vi "Collect_Info_updated.vi"(5 "HART ports":refnum<visa-resource-name>[](array[refnum]), 7 "485 Ports":refnum<visa-resource-name>[](array[refnum]), 10 "MODBUS Serial Parameters":T8={"Mode"=enum."RTU", "Default Slave Address"=111, "MODBUS timeout"=1000, "Baud Rate"=38400, "Parity"=0, "Flow Control"=0} {"Flow Control" items=["None", "XON/XOFF", "RTS/CTS", "XON/XOFF & RTS/CTS", "DTR/DSR", "XON/XOFF & DTR/DSR"]; "Parity" items=["None", "Odd", "Even", "Mark", "Space"]}) -> (1 "Read Completed":bool, 2 "Information":T9, 3 "Byte order":T2(ring))   [LabVIEW 2016]
uses:
  Controls/Flow Tube Material.ctl
  Controls/mass flow unit codes.ctl
  Controls/Density Unit codes.ctl
  Controls/Temperature units.ctl
  Controls/Flow direction codes.ctl
  Controls/Information_tab_type.ctl
  OPC Server/MODBUS/MODBUS parameters type.ctl
  <vilib>/DeviceNet/VIAPI/subVIs/DnetIntfConfig.ctl
  OPC Server/Typedef/Array_of_Comm_mode_and_address_types.ctl
  OPC Server/Typedef/Comm_mode_and_address_type.ctl
  OPC Server/Typedef/Comm_mode_type_combo.ctl
  types/Control_EXIT.ctl
  Controls/ctrlCollectInfoStates.ctl
  Controls/ctrlCollectInfoData.ctl
  OPC Server/Protocol Class/Protocol.lvclass
  OPC Server/Typedef/comm_variable_definition.ctl
  OPC Server/MASTER_OPC.ctl
  OPC Server/Typedef/event var.ctl
  OPC Server/Typedef/Comm ui action type.ctl
  OPC Server/Typedef/Comm_State_enum.ctl
  OPC Server/Typedef/state var.ctl
  <vilib>/Utility/miscctls.llb/LVPointTypeDef.ctl
  OPC Server/MODBUS/MODBUS Class/MODBUS.lvclass
  C:/Applications/Blackbox_US-Rabi--master/OPC Server/Protocol Class/Protocol.lvclass
  OPC Server/HART/HART Class/HART.lvclass
  OPC Server/Profibus/Profibus Class/Profibus.lvclass
  OPC Server/DeviceNET/DeviceNET Class/DeviceNET.lvclass
  OPC Server/Typedef/Protocol_enum_type.ctl
  <vilib>/DeviceNet/DeviceNetLIB.lvlib
panel:
  in  "Exit":T1
  in  "MDOT":string="H2O"
  in  "Meter inlet static pressure (psia)":dbl
  in  "Fluid":string="H2O"
  in  "Product code*":string
  in  "Order number":string
  in  "Status *":enum32{"As found", "As left"}(radio)
  in  "Ref meter serial number*":string
  in  "Technician Name*":string
  in  "Customer Address":string
  in  "Customer Name":string
  in  "Done":bool
  out "status":bool
  in  "Protocol selection\n(appended)":T3=[{"address"=111, "Mode"=0}, {"address"=0, "Mode"=2}] {"Mode" items=["MODBUS", "HART", ""]}
  in  "Interface Name":T6(ring)
  in  "DeviceNet Interface Configuration":T7={"interface MAC ID"=0, "baud rate"=enum."500000", "poll mode"=enum."Automatic"} {"interface MAC ID" max=63 step=1}
  in  "Profibus Baud rate":i32(listbox)=6
  in  "Profibus ResourceName":refnum<visa-resource-name>="PXI5::11::INSTR"
  in  "Read":bool
  in  "Test Comments":string
  out "Test date and time":string
  out "Meter Zero":string
  in  "Meter Nominal Flow Rate (kg/min)*":string
  in  "Meter Density Repeatability":string
  in  "Meter Density Accuracy":string
  in  "Meter Zero Stability (kg/min) *":string
  in  "Meter flow repeatability":string
  in  "Meter flow accuracy (%) *":string
  out "Frequency span":string
  out "Frequency flow rate":string
  out "Flow direction":T10 items=["Forward flow only", "Reverse flow only", "Bidirectiona flow", "Absolute forward/reverse", "Negate/Forward only", "Negate/Bidirectional"]
  out "Mass flow damping":string
  out "Mass flow cutoff":string
  out "Temperature Units":T11 items=["Degrees Celsius"=32, "Degrees Fahrenheit"=33, "Degrees Rankine"=34, "Degrees Kelvin"=35, ""=0]
  out "Density units":T12 items=["Specific gravity units"=90, "Grams/cubic centimeter"=91, "Kg/cubic meter"=92, "Pounds/US gallon"=93, "Pounds/cubic foot"=94, "Grams/milliliter"=95, "Kg/liter"=96, "Pounds/cubic inch"=98, "Short tons/cubic yard"=99, "Degrees Baume (heavy)"=102, "Degrees Baume (light)"=103, "Degrees API"=104]
  out "Mass flow units":T13 items=["Grams/second"=70, "Grams/minute"=71, "Grams/hour"=72, "Kg/second"=73, "Kg/minute"=74, "Kg/hour"=75, "Kg/day"=76, "Metric tons/minute"=77, "Metric tons/hour"=78, "Metric tons/day"=79, "Pounds/second"=80, "Pounds/minute"=81, "Pounds/hour"=82, "Pounds/day"=83, "Short tons/minute"=84, "Short tons/hour"=85, "Short tons/day"=86, "Long tons/hour"=87, "Long tons/day"=88, "Special"=253]
  out "Transmitter Model":string
  in  "Sensor Model #":string
  in  "Transmitter Serial Number":string
  out "Density Temp Coeff":string
  out "FD":string
  out "K2":string
  out "K1":string
  out "D2":string
  out "D1":string
  out "FCF":string
  in  "Temp Rating":string
  in  "Pressure Rating":string
  out "Sensor Serial Number":string
  out "Flow Tube Material":T14 items=["Hastelloy C-22"=3, "Monel"=4, "Tantalum"=5, "Titanium"=6, "316L Stainless Steel"=19, "Inconel"=23, "Unknown"=252, "Special"=253]
  in  "Size":string
  # "Customer Information"
  # "*Required"
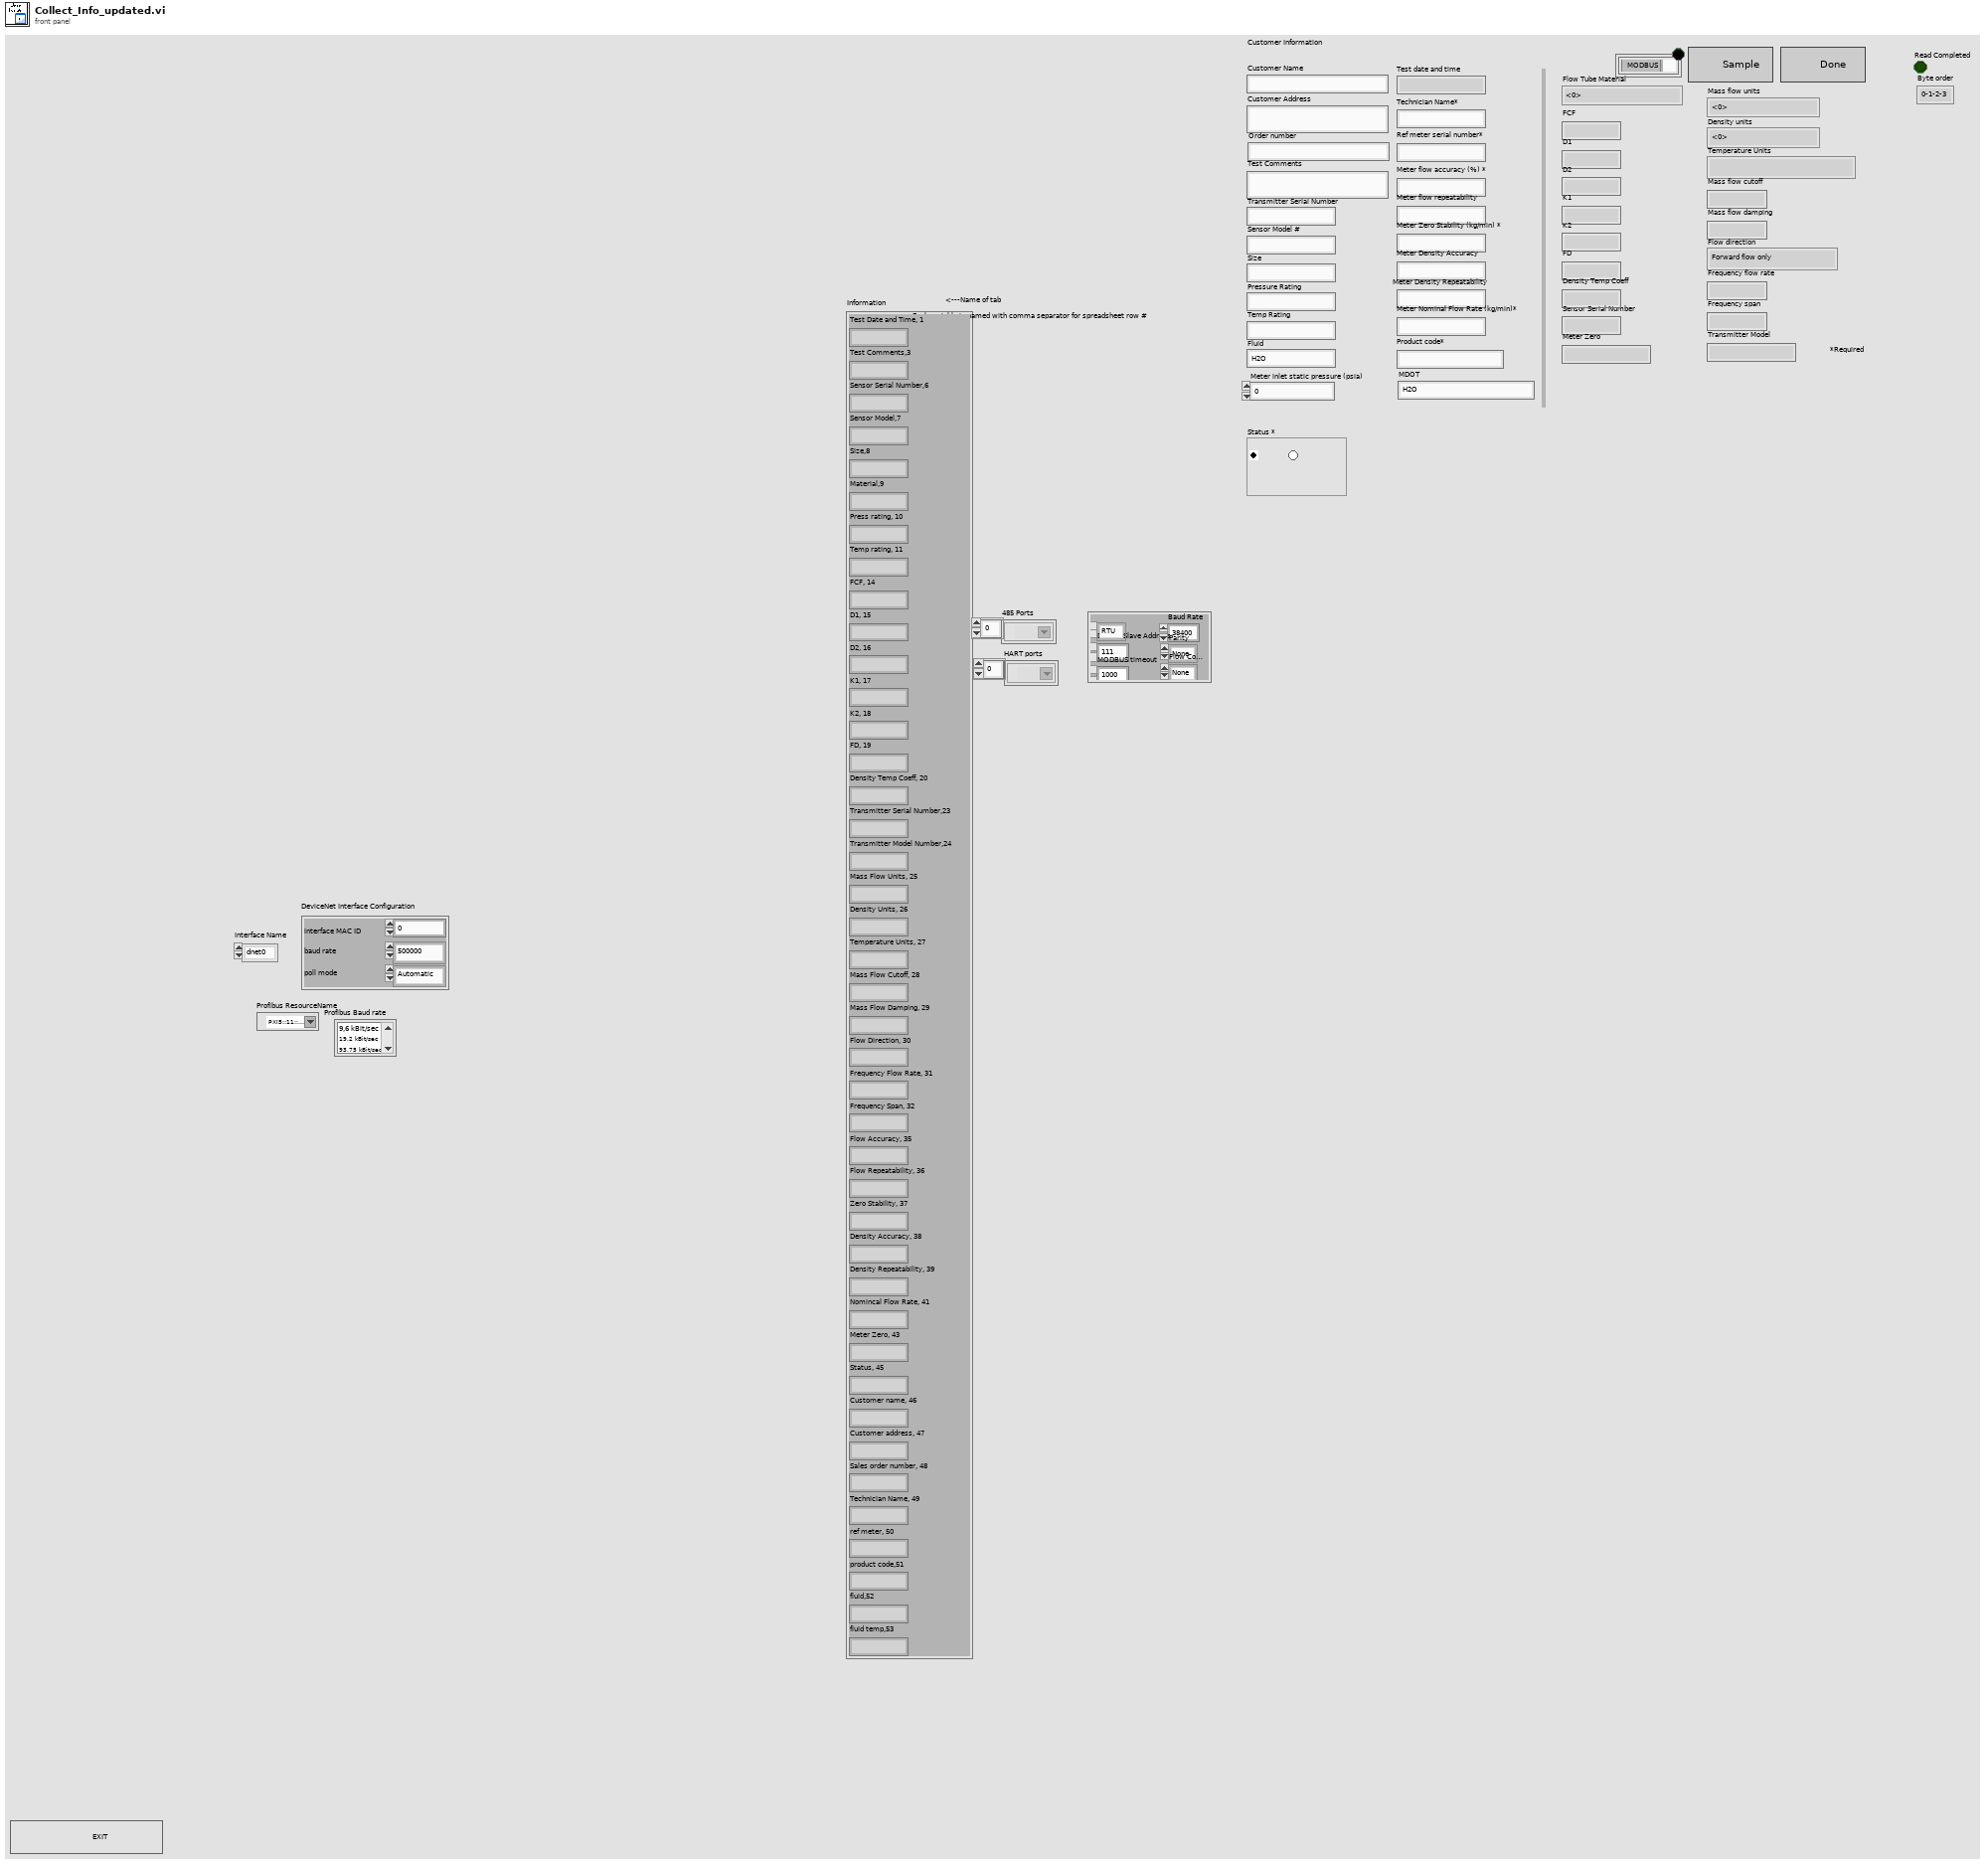
[diagram p1: front panel]
types:
  T1 = typedef "Control_EXIT.ctl" = bool
  T2 = enum16{"0-1-2-3", "2-3-0-1", "1-0-3-2", "3-2-1-0"}
  T3 = typedef "Array_of_Comm_mode_and_address_types.ctl" = T4[]
  T4 = typedef "Comm_mode_and_address_type.ctl" = cluster{"address":i32, "Mode":T5}
  T5 = typedef "Comm_mode_type_combo.ctl" = u16
  T6 = enum16{"dnet0", "dnet1", "dnet2", "dnet3", "dnet4", "dnet5", "dnet6", "dnet7", "dnet8", "dnet9", "dnet10", "dnet11", "dnet12", "dnet13", "dnet14", "dnet15", "dnet16", "dnet17", "dnet18", "dnet19", "dnet20", "dnet21", "dnet22", "dnet23", "dnet24", "dnet25", "dnet26", "dnet27", "dnet28", "dnet29", "dnet30", "dnet31"}
  T7 = typedef "DeviceNetLIB.lvlib/DnetIntfConfig.ctl" = cluster{"interface MAC ID":u32, "baud rate":enum32{"125000", "250000", "500000"}, "poll mode":enum32{"Automatic", "Scanned", "Individual"}}
  T8 = typedef "MODBUS parameters type.ctl" = cluster{"Mode":enum16{"RTU", "ASCII"}, "Default Slave Address":u8, "MODBUS timeout":u32, "Baud Rate":u32, "Parity":u16, "Flow Control":u16}
  T9 = typedef "Information_tab_type.ctl" = cluster{"Test Date and Time, 1":string, "Test Comments,3":string, "Sensor Serial Number,6":string, "Sensor Model,7":string, "Size,8":string, "Material,9":string, "Press rating, 10":string, "Temp rating, 11":string, "FCF, 14":string, "D1, 15":string, "D2, 16":string, "K1, 17":string, "K2, 18":string, "FD, 19":string, "Density Temp Coeff, 20":string, "Transmitter Serial Number,23":string, "Transmitter Model Number,24":string, "Mass Flow Units, 25":string, "Density Units, 26":string, "Temperature Units, 27":string, "Mass Flow Cutoff, 28":string, "Mass Flow Damping, 29":string, "Flow Direction, 30":string, "Frequency Flow Rate, 31":string, "Frequency Span, 32":string, "Flow Accuracy, 35":string, "Flow Repeatability, 36":string, "Zero Stability, 37":string, "Density Accuracy, 38":string, "Density Repeatability, 39":string, "Nomincal Flow Rate, 41":string, "Meter Zero, 43":string, "Status, 45":string, "Customer name, 46":string, "Customer address, 47":string, "Sales order number, 48":string, "Technician Name, 49":string, "ref meter, 50":string, "product code,51":string, "fluid,52":string, "fluid temp,53":string}
  T10 = typedef "Flow direction codes.ctl" = u16
  T11 = typedef "Temperature units.ctl" = u16
  T12 = typedef "Density Unit codes.ctl" = u16
  T13 = typedef "mass flow unit codes.ctl" = u16
  T14 = typedef "Flow Tube Material.ctl" = u16
  T15 = typedef "ctrlCollectInfoData.ctl" = cluster{"HART ports":refnum<visa-resource-name>[], "485 ports":refnum<visa-resource-name>[], "Byte order":enum16{"0-1-2-3", "2-3-0-1", "1-0-3-2", "3-2-1-0"}, "Read Complete?":bool, "ProtocolRef":refnum<vi>, "Data path":path, "ProtocolArray":refnum<class "Protocol.lvclass">[], "Protocol":refnum<class "Protocol.lvclass">, "Comm variable definitions":T16[], "Information":T9}
  T16 = typedef "comm_variable_definition.ctl" = cluster{"General Parameter name":string, "MODBUS Register":i32, "Profibus":cluster{"Friendly name":string, "PA":cluster{"Slot":i32, "Index":i32}, "DP":cluster{"Slot":i32, "Index":i32}, "Tag":string}, "Fieldbus":cluster{"Parameter name":string, "Fieldbus Block":string, "Fieldbus Tag":string}, "data type":enum16{"float", "UINT", "UINT32", "STRING"}, "DeviceNET":cluster{"ClassId":u16, "InstanceId":u16, "AttributeId":u8}, "Cluster":T4, "Length":i32}
  T17 = typedef "ctrlCollectInfoStates.ctl" = enum16{"WaitforEvents", "Init", "Read-Protocol", "Read-CommInfo", "Read-ByteOrder", "Read-FlowTubeMaterial", "Read-FlowCalibFactor", "Read-D1", "Read-D2", "Read-K1", "Read-K2", "Read-FD", "Read-DenTempCoeff", "Read-Srno", "Read-MassFlowUnits", "Read-DensityUnits", "Read-TempUnits", "Read-FlowCutoff", "Read-MassFlowDamping", "Read-FlowDirection", "Read-FreqFlowRate", "Read-FreqSpan", "Read-TransmitterModel", "Read-MeterZero", "ReadComplete", "Done&Close"}
  T18 = typedef "LVPointTypeDef.ctl" = cluster{"Horizontal":i16, "Vertical":i16}
  T19 = typedef "MASTER_OPC.ctl" = cluster{"Main event var":refnum<user-event>, "VIRef":refnum<vi>, "Data path":path, "Reads":i32, "total number of UUT":i32, "FF refnum":cluster{"Handle1":u32, "Handle2":u32}, "FF device id list":string[], "MODBUS resource name":refnum<visa-resource-name>, "MODBUS Serial Parameters":cluster{"Mode":enum16{"RTU", "ASCII"}, "Default Slave Address":u8, "MODBUS timeout":u32, "Baud Rate":u32, "Parity":u16, "Flow Control":u16}, "Profibus resource name":refnum<visa-resource-name>, "Profibus Communication ref.:":u8, "HART resource name":refnum<visa-resource-name>, "HART long addresses (array)":u8[][], "Comm relay session":refnum<k15>, "Comm UI event":refnum<user-event>, "Write Interval (s)":dbl, "DMM_QUEUE":refnum<queue>, "POWER_QUEUE":refnum<queue>, "\nTHERM_QUEUE":refnum<queue>, "\nCOMM_QUEUE":refnum<queue>, "TIMING_QUEUE":refnum<queue>, "MAIN_QUEUE":refnum<queue>, "Log path":path}
  T20 = typedef "Protocol_enum_type.ctl" = enum16{"None", "MODBUS", "HART", "Fieldbus", "Profibus DP", "Profibus PA", "DeviceNET", "USB"}
  T21 = typedef "CS_PB_DPV1_MSAC2_InitiateReqData.ctl" = cluster{"Communication ref.:":u8, "Send timeout:":u16, "Feat. supp. 1:":u8, "Feat. supp. 2:":u8, "Profile feat. supp. 1:":u8, "Profile feat. supp. 2:":u8, "Profile ID number:":u16, "Addional address parameter":cluster{"S-Type":bool, "S-Length:":u8, "D-Type":bool, "D-Length:":u8, "Data:":u8[]}}
  T22 = cluster{"U16":u16, "U32":u32, "float":sgl, "string":string}
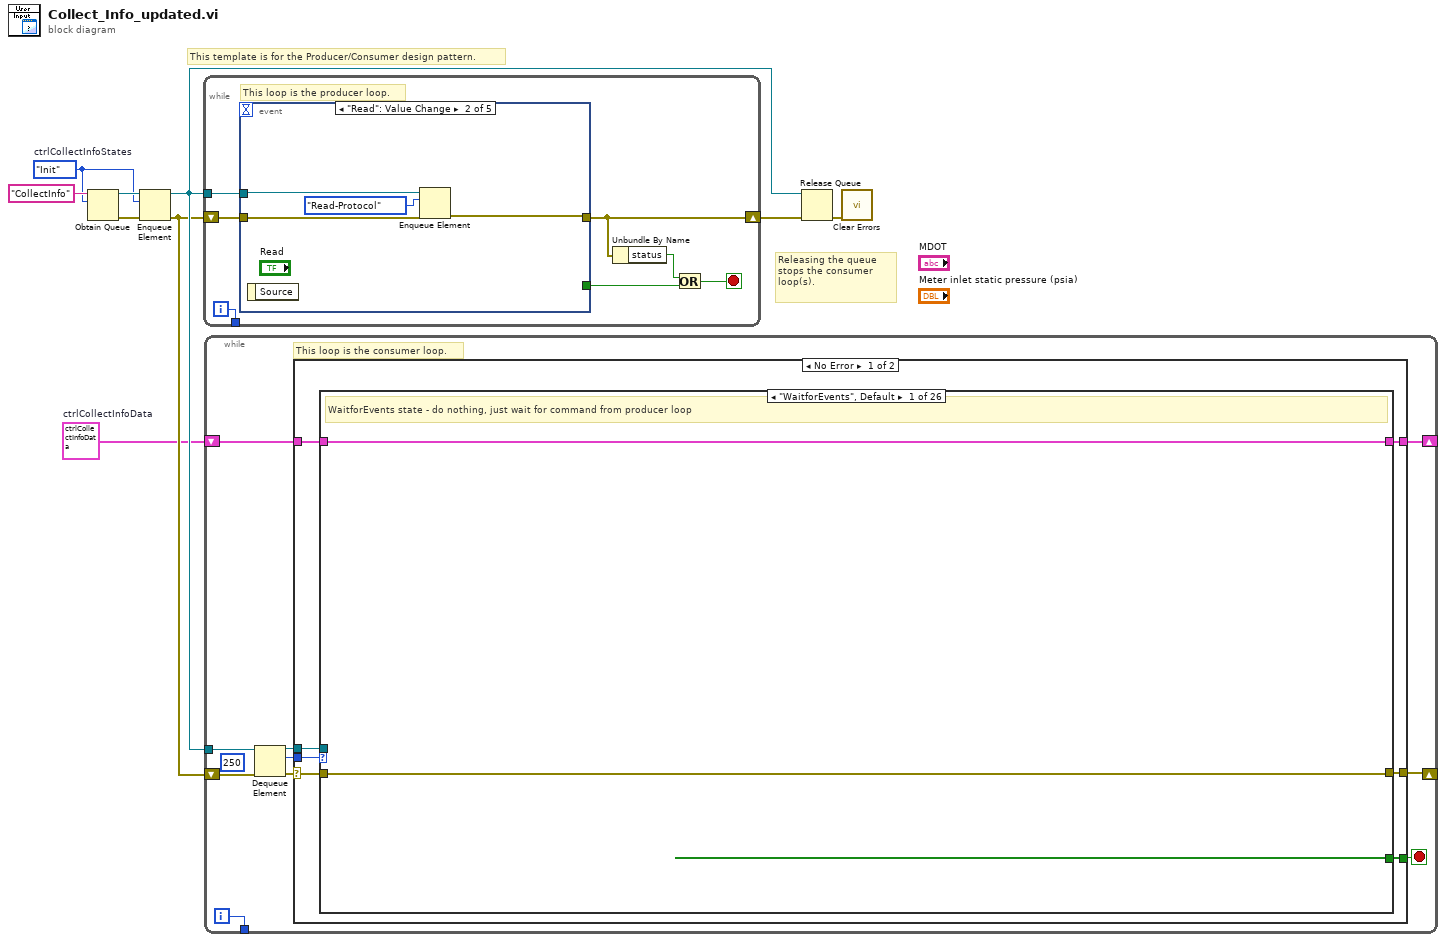
[diagram p0: block diagram]
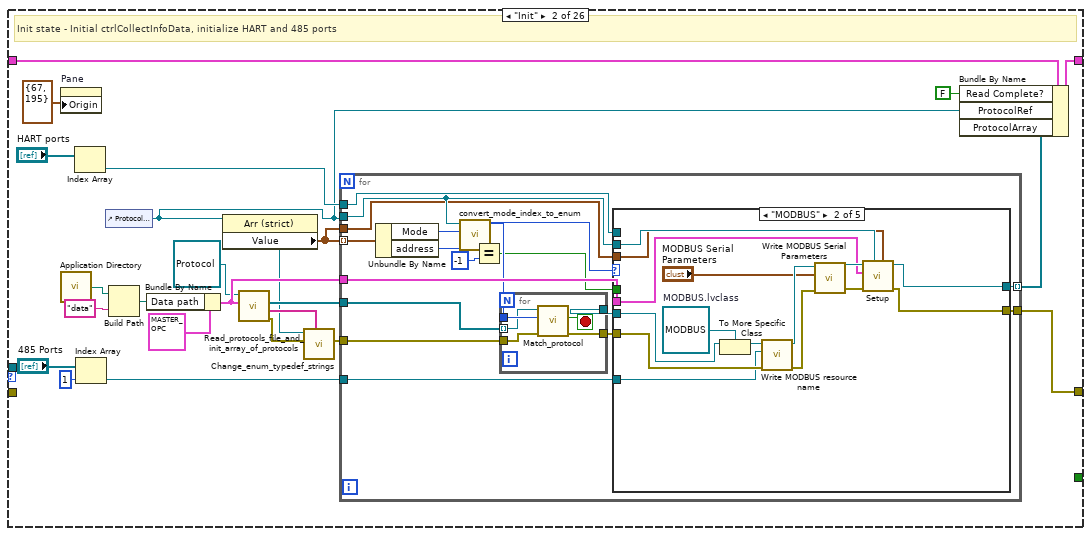
[diagram p2: hidden frame]
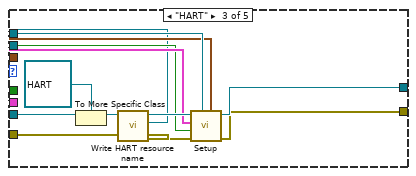
[diagram p4: hidden frame]
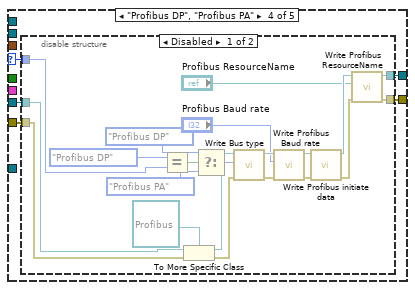
[diagram p5: hidden frame]
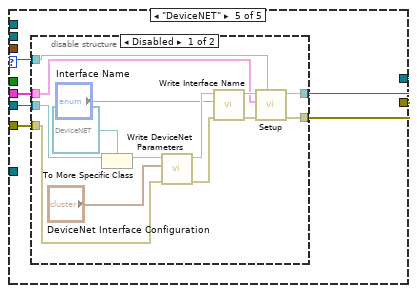
[diagram p7: hidden frame]
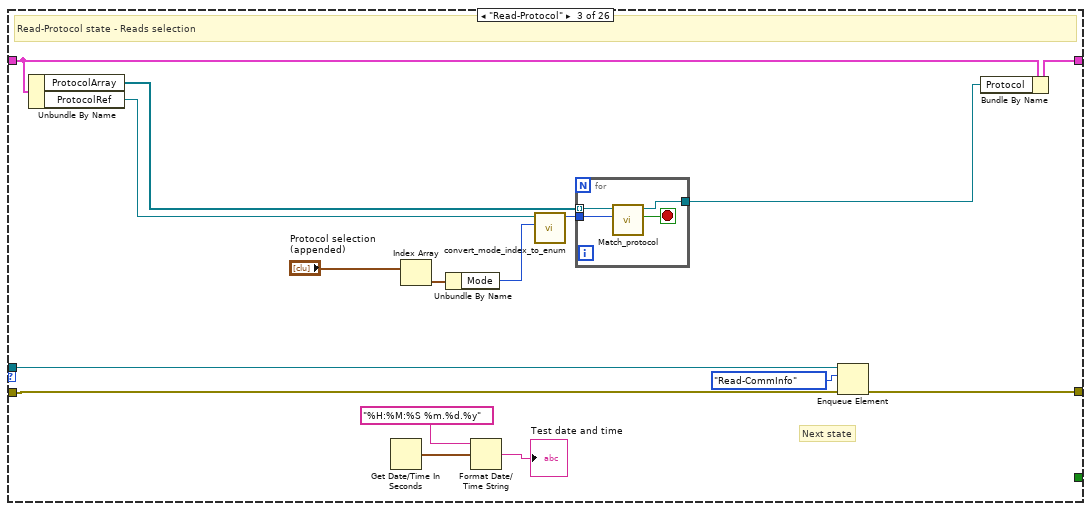
[diagram p9: hidden frame]
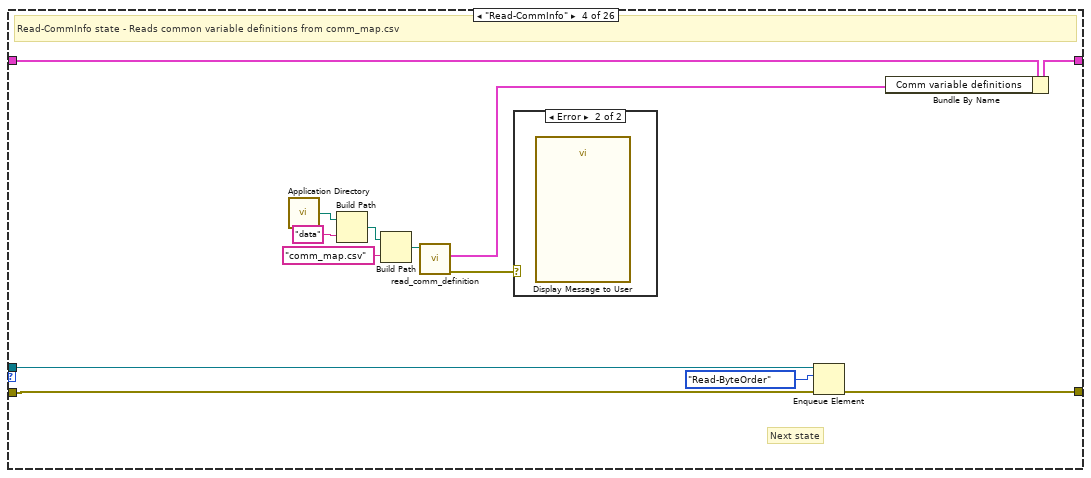
[diagram p10: hidden frame]
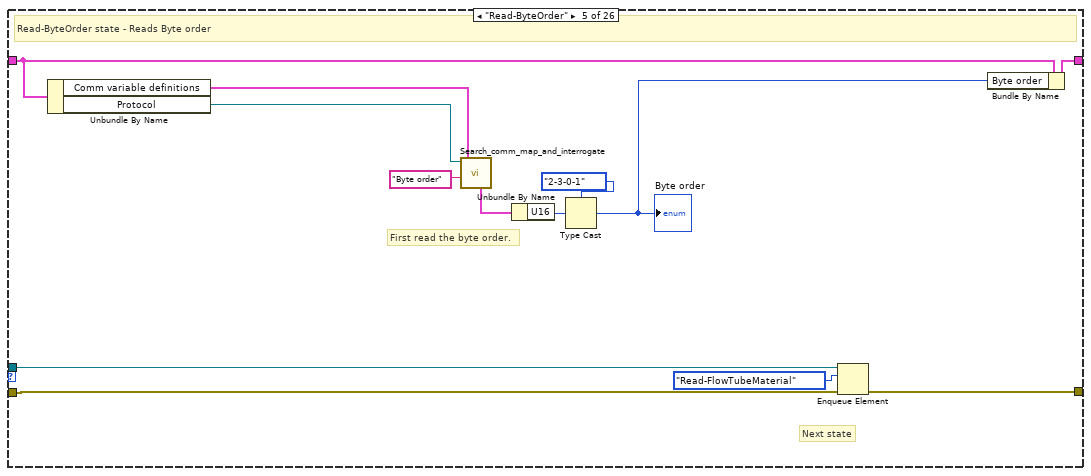
[diagram p12: hidden frame]
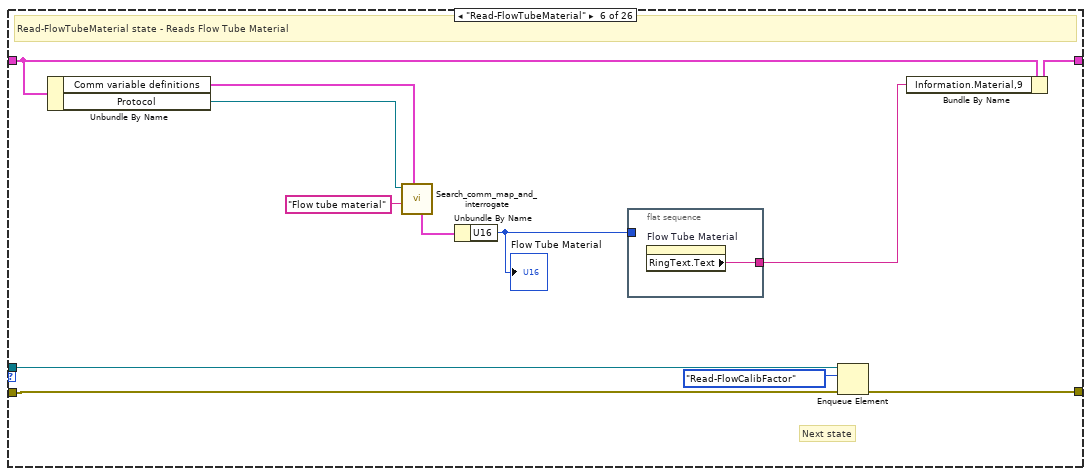
[diagram p13: hidden frame]
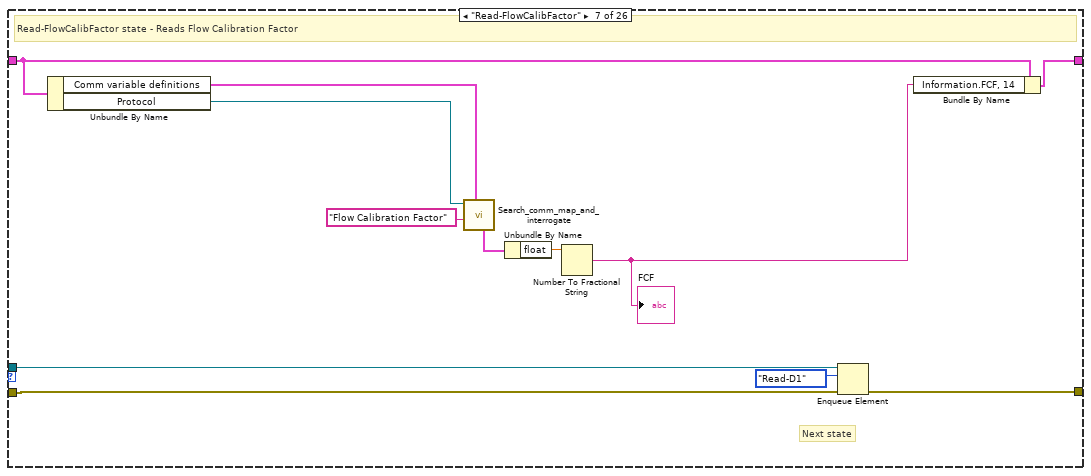
[diagram p14: hidden frame]
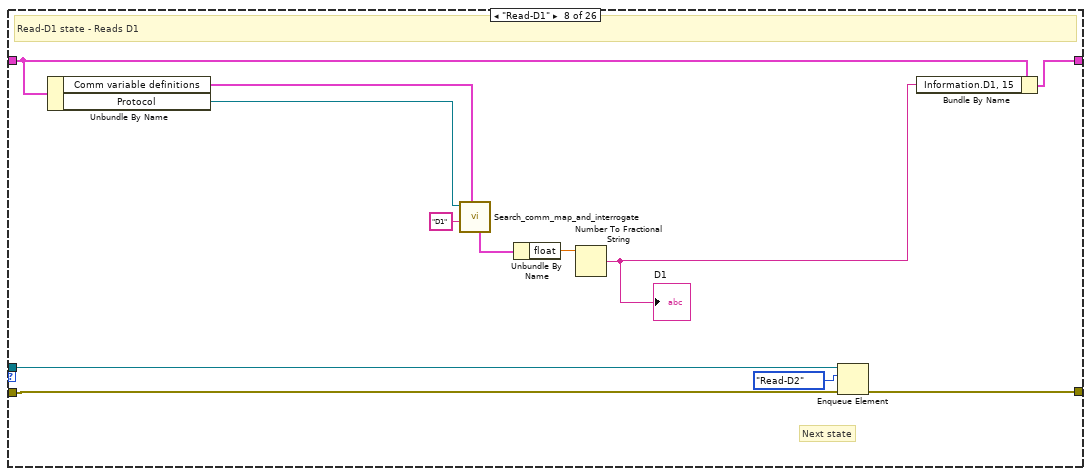
[diagram p15: hidden frame]
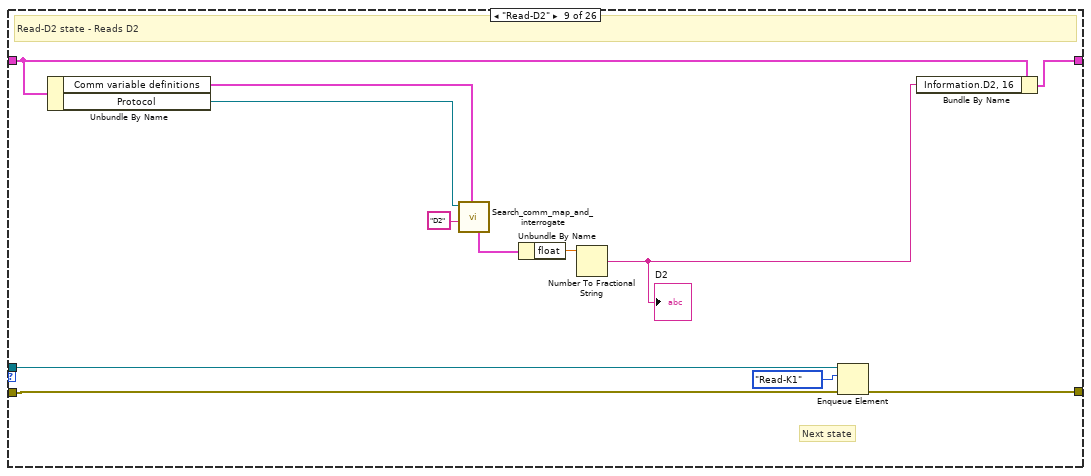
[diagram p16: hidden frame]
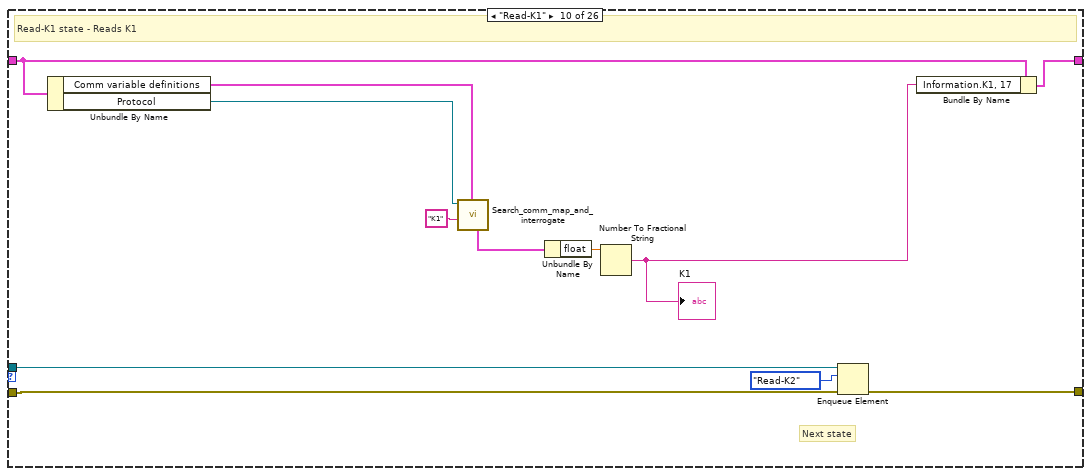
[diagram p17: hidden frame]
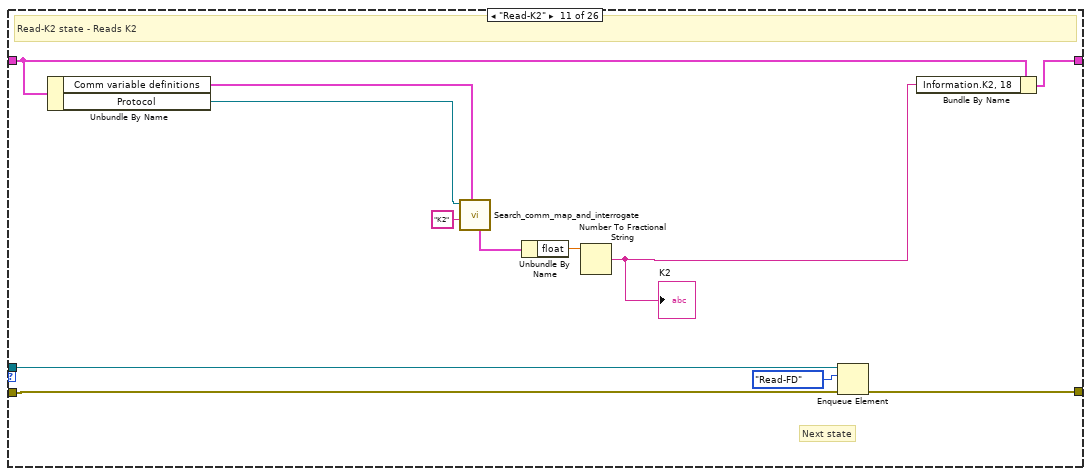
[diagram p18: hidden frame]
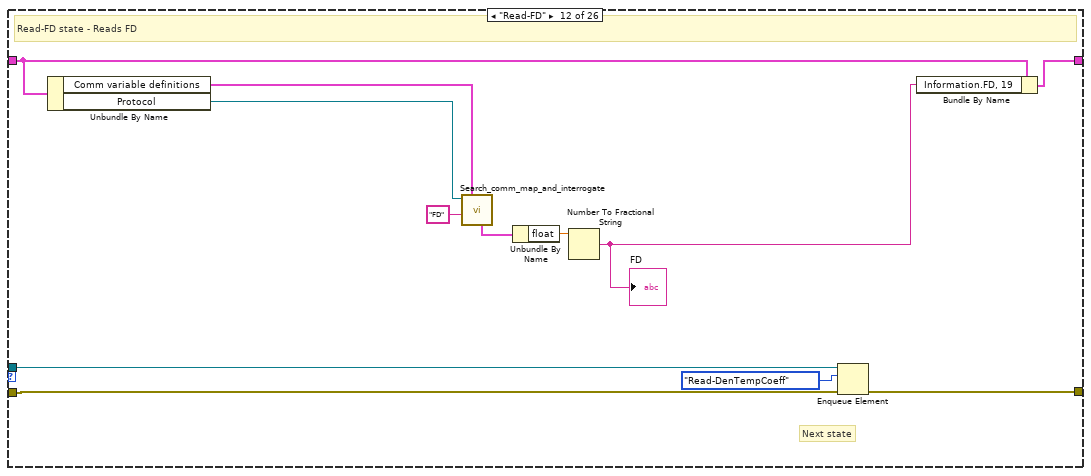
[diagram p19: hidden frame]
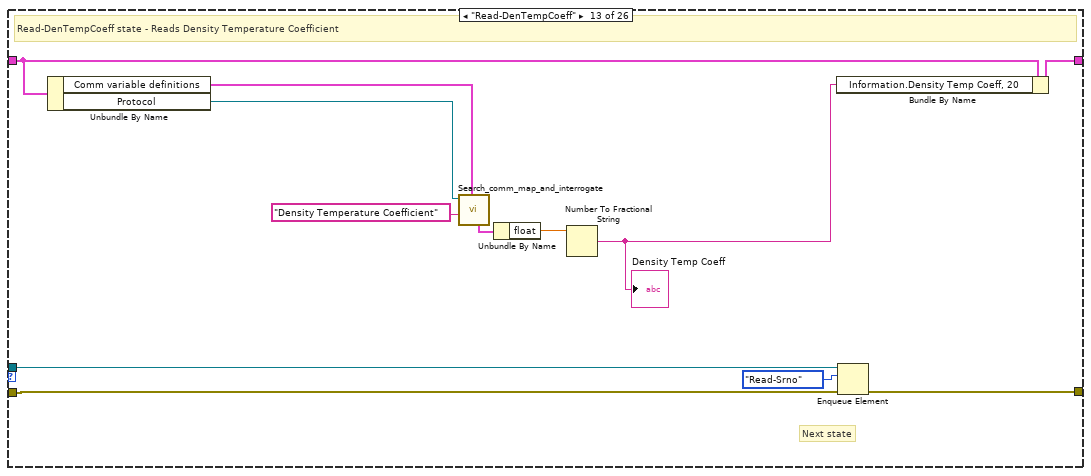
[diagram p20: hidden frame]
diagram:
  w1 = T15 {"HART ports"=[], "485 ports"=[], "Byte order"=enum."0-1-2-3", "Read Complete?"=FALSE, "ProtocolRef"=refnum, "Data path"=path "", "ProtocolArray"=[], "Protocol"=refnum, "Comm variable definitions"=[], "Information"={"Test Date and Time, 1"="", "Test Comments,3"="", "Sensor Serial Number,6"="", "Sensor Model,7"="", "Size,8"="", "Material,9"="", "Press rating, 10"="", "Temp rating, 11"="", "FCF, 14"="", "D1, 15"="", "D2, 16"="", "K1, 17"="", "K2, 18"="", "FD, 19"="", "Density Temp Coeff, 20"="", "Transmitter Serial Number,23"="", "Transmitter Model Number,24"="", "Mass Flow Units, 25"="", "Density Units, 26"="", "Temperature Units, 27"="", "Mass Flow Cutoff, 28"="", "Mass Flow Damping, 29"="", "Flow Direction, 30"="", "Frequency Flow Rate, 31"="", "Frequency Span, 32"="", "Flow Accuracy, 35"="", "Flow Repeatability, 36"="", "Zero Stability, 37"="", "Density Accuracy, 38"="", "Density Repeatability, 39"="", "Nomincal Flow Rate, 41"="", "Meter Zero, 43"="", "Status, 45"="", "Customer name, 46"="", "Customer address, 47"="", "Sales order number, 48"="", "Technician Name, 49"="", "ref meter, 50"="", "product code,51"="", "fluid,52"="", "fluid temp,53"=""}}  # ctrlCollectInfoData
  w2 = ctrlCollectInfoStates."Init"  # ctrlCollectInfoStates
  # "This template is for the Producer/Consumer design pattern."
  # "Releasing the queue stops the consumer loop(s)."
  n1 = Obtain Queue(name (unnamed)="CollectInfo", element data type=w2) -> (queue out=w9:refnum<queue>, error out=w6:errorcluster)  [unwired: 3 in, 1 out]
  n2 = Enqueue Element(queue=w9, element=w2, error in (no error)=w6) -> (queue out=w4:refnum<queue>, error out=w3:errorcluster)  [unwired: 1 in, 1 out]
  n3 = while {
    tunnel: w4 -> [w16]
    tunnel: [w15] -> _
    shift-right: [w11] -> w5
    shift-left: w3 -> [w14]
    i -> [w15]
    stop <- w12 stop-if-true
    # "This loop is the producer loop."
    n4 = event shown="[1] \"Read\": Value Change" {
      selector: _ -> [_ _ _ _ _]
      dyn-events: _ -> [_ _ _ _ _]
      timeout: _ -> [_ _ _ _ _]
      tunnel: w16 -> [w17 w22 w26 _ _]
      tunnel: w14 -> [w20 w24 w29 w34 w39]
      tunnel: [w19 w23 w28 w34 w39] -> w11
      tunnel: [_ _ TRUE ("T button?") w31 w35] -> w10
      event Value Change {
        n5 = event-data() -> ()  [unwired: 1 in, 1 out]
        n6 = Enqueue Element(queue=w17, element=ctrlCollectInfoStates."Init" ("ctrlCollectInfoStates"), error in (no error)=w20) -> (error out=w19:errorcluster)  [unwired: 1 in, 2 out]
      }
      event "Read": Value Change {
        n7 = event-data() -> ()  [unwired: 1 in, 1 out]
        n8 = Enqueue Element(queue=w22, element=ctrlCollectInfoStates."Read-Protocol" ("ctrlCollectInfoStates"), error in (no error)=w24) -> (error out=w23:errorcluster)  [unwired: 1 in, 2 out]
      }
      event "Done": Value Change {
        n9 = event-data() -> ()  [unwired: 1 in, 1 out]
        n10 = Enqueue Element(queue=w26, element=ctrlCollectInfoStates."Done&Close" ("ctrlCollectInfoStates"), error in (no error)=w29) -> (error out=w28:errorcluster)  [unwired: 1 in, 2 out]
      }
      event Panel Close? {
        (unwired) "Cancel" ("F button name (\"Cancel\")")
        n11 = event-data() -> ()  [unwired: 1 in, 1 out]
        n12 = Two Button Dialog(message="Quitting will Abort all running program\nAre you sure you want to exit?", 2:"Quit" ("T button name (\"OK\")")) -> (T button?=w31:bool)  [unwired: 1 in]
        n13 = Not(x=w31) -> (.not. x?=w30:bool)
        n14 = event-data("Discard?"=w30) -> ()  [unwired: 1 in, 1 out]
      }
      event Value Change {
        n15 = event-data() -> ()  [unwired: 1 in, 1 out]
        n16 = Two Button Dialog(message="Quitting will Abort all running program\nAre you sure you want to exit?", 1:"Cancel" ("F button name (\"Cancel\")"), 2:"Quit" ("T button name (\"OK\")")) -> (T button?=w35:bool)
      }
    }
    n17 = Unbundle By Name(w11) -> ("status"=w13:bool)
    n18 = Or(x=w13, y=w10) -> (x .or. y?=w12:bool)
  }
  n19 = while {
    tunnel: w4 -> [w49]
    shift-right: [w44] -> _
    shift-left: w1 -> [w45]
    shift-right: [w41] -> _
    shift-left: w3 -> [w42]
    tunnel: [w40] -> _
    i -> [w40]
    stop <- w46 stop-if-true
    (unwired) 250 ("timeout in ms (-1)")
    # "This loop is the consumer loop."
    n20 = Dequeue Element(queue=w49, error in (no error)=w42) -> (queue out=w43:refnum<queue>, element=w47:T17, error out=w48:errorcluster)  [unwired: 1 in, 1 out]
    n21 = case shown="No Error" w48 {
      selector: w48 -> [w51 w503]
      tunnel: w47 -> [w54 _]
      tunnel: [w50 FALSE] -> w46
      tunnel: w45 -> [w55 w504]
      tunnel: [w56 w504] -> w44
      tunnel: w43 -> [w53 _]
      tunnel: [w52 w502] -> w41
      frame No Error {
        n22 = case shown="\"WaitforEvents\", Default" w54 {
          tunnel: [w57 w69 w197 w207 w217 w239 w252 w264 w276 w288 w300 w312 w324 w336 w348 w361 w374 w387 w399 w411 w424 w436 w448 w462 w469 w473] -> w56
          tunnel: w55 -> [w57 w70 w189 w208 w218 w235 w248 w260 w272 w284 w296 w308 w320 w332 w344 w357 w370 w383 w395 w407 w420 w432 w444 w457 w464 w474]
          tunnel: w53 -> [_ _ w196 w205 w227 w238 w251 w263 w275 w287 w299 w311 w323 w335 w347 w360 w373 w386 w398 w410 w423 w435 w447 w461 w468 _]
          tunnel: [w58 w61 w194 w203 w225 w236 w249 w261 w273 w285 w297 w309 w321 w333 w345 w358 w371 w384 w396 w408 w421 w433 w445 w459 w466 w471] -> w52
          tunnel: w51 -> [w58 _ w195 w204 w226 w237 w250 w262 w274 w286 w298 w310 w322 w334 w346 w359 w372 w385 w397 w409 w422 w434 w446 w460 w467 w471]
          tunnel: [_ _ _ _ _ _ _ _ _ _ _ _ _ _ _ _ _ _ _ _ _ _ _ _ _ TRUE] -> w50
          frame "WaitforEvents", Default {
            # "WaitforEvents state - do nothing, just wait for command from producer loop"
          }
          frame "Init" {
            # "Init state - Initial ctrlCollectInfoData, initialize HART and 485 ports"
            n23 = property on="Pane" class="Pane"("Origin"=T18 {"Horizontal"=67, "Vertical"=195}) -> ()  [unwired: 2 in, 2 out]
            n24 = call <vilib>:"Application Directory.vi"() -> ("Application Directory"=w78:path)
            n25 = Index Array(array="HART ports") -> (element=w64:refnum<visa-resource-name>)  [unwired: 1 in]
            n26 = Index Array(array="485 Ports", index=1) -> (element=w63:refnum<visa-resource-name>)
            n27 = control-ref of="Protocol selection\n(appended)"() -> (w62:refnum<vi>)
            n28 = Build Path(base path=w78, name or relative path="data") -> (appended path=w80:path)
            n29 = Bundle By Name(cluster=T19 {"Main event var"=refnum, "VIRef"=refnum, "Data path"=path "", "Reads"=0, "total number of UUT"=0, "FF refnum"={"Handle1"=0, "Handle2"=0}, "FF device id list"=[], "MODBUS resource name"="", "MODBUS Serial Parameters"={"Mode"=enum."RTU", "Default Slave Address"=0, "MODBUS timeout"=0, "Baud Rate"=0, "Parity"=0, "Flow Control"=0}, "Profibus resource name"="", "Profibus Communication ref.:"=0, "HART resource name"="", "HART long addresses (array)"=[], "Comm relay session"="", "Comm UI event"=refnum, "Write Interval (s)"=5.0, "DMM_QUEUE"=refnum, "POWER_QUEUE"=refnum, "\nTHERM_QUEUE"=refnum, "\nCOMM_QUEUE"=refnum, "TIMING_QUEUE"=refnum, "MAIN_QUEUE"=refnum, "Log path"=path ""} ("Comm master cluster"), "Data path"=w80) -> (w81:T19)
            n30 = property class="Arr (strict)"(reference=w62) -> ("Value"=w71:T3)  [unwired: 1 in, 2 out]
            n31 = call-dynamic "Read_protocols_file_and_init_array_of_protocols.vi"("Comm master cluster"=w81, "Protocol in"=refnum<class "Protocol.lvclass"> refnum) -> ("error out"=w75:errorcluster, "Array of configured protocols"=w74:string[], "Array of Protocols out"=w73:refnum<class "Protocol.lvclass">[])  [unwired: 6 in, 1 out]
            n32 = call "Change_enum_typedef_strings.vi"("Strings []"=w74, "error in (no error)"=w75, "protocol selection ref"=w62) -> ("error out"=w76:errorcluster)  [unwired: 8 in]
            n33 = for {
              tunnel: w73 -> [w92]
              tunnel: [w98] -> w68 mode=indexing
              tunnel: [w97] -> w61
              tunnel: w62 -> [w95]
              tunnel: w76 -> [w89]
              tunnel: w81 -> [w96]
              tunnel: w71 -> [w94] mode=indexing
              tunnel: w71 -> [w84]
              tunnel: w64 -> [w83]
              tunnel: w63 -> [w82]
              n34 = Unbundle By Name(w94) -> ("Mode"=w93:T5, "address"=w87:i32)
              n35 = call "convert_mode_index_to_enum.vi"("index"=w93, "CtlRef"=w95) -> ("Protocol enum"=w88:T20)  [unwired: 6 in, 3 out]
              n36 = Equal?(x=w87, y=-1) -> (x = y?=w85:bool)
              n37 = for {
                tunnel: [w104] -> w91
                tunnel: [w102] -> w90
                tunnel: w88 -> [w101]
                tunnel: w92 -> [w100] mode=indexing
                tunnel: w89 -> [w99]
                stop <- w103 stop-if-true
                n38 = call-dynamic "Match_protocol.vi"("error in (no error)"=w99, "Protocol type"=w101, "Protocol in"=w100) -> ("error out"=w102:errorcluster, "Match"=w103:bool, "Protocol out"=w104:refnum<class "Protocol.lvclass">)  [unwired: 6 in]
              }
              n39 = case shown="\"MODBUS\"" w88 {
                selector: w88 -> [_ _ _ w136 _]
                tunnel: w91 -> [w106 w121 w134 w139 w167]
                tunnel: [w106 w119 w130 w135 w166] -> w98
                tunnel: [w105 w112 w127 w138 w165] -> w97
                tunnel: w90 -> [w105 w111 w132 w137 w164]
                tunnel: w96 -> [_ w110 w129 _ w163]
                tunnel: w95 -> [_ w109 w126 _ w162]
                tunnel: w85 -> [_ _ w124 _ _]
                tunnel: w84 -> [_ w108 w123 _ _]
                tunnel: w83 -> [_ _ w122 _ _]
                tunnel: w82 -> [_ w107 _ _ _]
                frame "None", Default {
                }
                frame "MODBUS" {
                  w120 = refnum<class "MODBUS.lvclass"> refnum  # MODBUS.lvclass
                  n40 = To More Specific Class(target class=w120, reference=w121) -> (specific class reference=w118:refnum<class "MODBUS.lvclass">)  [unwired: 1 in, 1 out]
                  n41 = call-dynamic "Write MODBUS resource name.vi"("error in (no error)"=w111, "MODBUS resource name"=w107, "MODBUS in"=w118) -> ("error out"=w117:errorcluster, "MODBUS out"=w116:refnum<class "MODBUS.lvclass">)  [unwired: 7 in]
                  n42 = call-dynamic "Write MODBUS Serial Parameters.vi"("error in (no error)"=w117, "MODBUS Serial Parameters"="MODBUS Serial Parameters", "MODBUS in"=w116) -> ("error out"=w113:errorcluster, "MODBUS out"=w114:refnum<class "MODBUS.lvclass">)  [unwired: 7 in]
                  n43 = call-dynamic "Setup.vi"("Protocol selection\n(appended)"=w108, "protocol selection ref"=w109, "error in (no error)"=w113, "Comm master cluster in"=w110, "MODBUS in"=w114) -> ("error out"=w112:errorcluster, "MODBUS out"=w119:refnum<class "MODBUS.lvclass">)  [unwired: 5 in]
                }
                frame "HART" {
                  n44 = To More Specific Class(target class=refnum<class "HART.lvclass"> refnum ("HART.lvclass"), reference=w134) -> (specific class reference=w133:refnum<class "HART.lvclass">)  [unwired: 1 in, 1 out]
                  n45 = call-dynamic "Write HART resource name.vi"("error in (no error)"=w132, "HART resource name"=w122, "HART in"=w133) -> ("error out"=w128:errorcluster, "HART out"=w131:refnum<class "HART.lvclass">)  [unwired: 7 in]
                  n46 = call-dynamic "Setup.vi"("Protocol selection\n(appended)"=w123, "protocol selection ref"=w126, "error in (no error)"=w128, "search"=w124, "Comm master cluster in"=w129, "HART in"=w131) -> ("error out"=w127:errorcluster, "HART out"=w130:refnum<class "HART.lvclass">)  [unwired: 4 in]
                }
                frame "Profibus DP", "Profibus PA" {
                  n47 = disable-structure shown="Disabled" {
                    disable-tunnel: w139 -> [w160 _]
                    disable-tunnel: [w156 _] -> w138
                    disable-tunnel: w137 -> [w150 _]
                    disable-tunnel: w136 -> [w148 _]
                    disable-tunnel: [w140 _] -> w135
                    frame Disabled {
                      n48 = Equal?(x=Protocol_enum_type."Profibus DP" ("Protocols"), y=w148) -> (x = y?=w147:bool)
                      n49 = To More Specific Class(target class=refnum<class "Profibus.lvclass"> refnum ("Profibus.lvclass"), reference=w160, error in=w150) -> (specific class reference=w152:refnum<class "Profibus.lvclass">, error out=w151:errorcluster)
                      n50 = Select(t=enum16{"Profibus DP", "Profibus PA"}."Profibus DP" ("Bus type"), s=w147, f=enum16{"Profibus DP", "Profibus PA"}."Profibus PA" ("Bus type")) -> (s? t:f=w144:enum16{"Profibus DP", "Profibus PA"})
                      n51 = call-dynamic "Write Bus type.vi"("error in (no error)"=w151, "Bus type"=w144, "Profibus in"=w152) -> ("error out"=w159:errorcluster, "Profibus out"=w155:refnum<class "Profibus.lvclass">)  [unwired: 7 in]
                      n52 = call-dynamic "Write Profibus Baud rate.vi"("error in (no error)"=w159, "Profibus Baud rate"="Profibus Baud rate", "Profibus in"=w155) -> ("error out"=w158:errorcluster, "Profibus out"=w154:refnum<class "Profibus.lvclass">)  [unwired: 7 in]
                      n53 = call-dynamic "Write Profibus initiate data.vi"("error in (no error)"=w158, "Profibus in"=w154) -> ("error out"=w157:errorcluster, "Profibus out"=w153:refnum<class "Profibus.lvclass">, "Initiate data"=w142:T21)  [unwired: 7 in]
                      n54 = call-dynamic "Write Profibus ResourceName.vi"("error in (no error)"=w157, "Profibus ResourceName"="Profibus ResourceName", "Profibus in"=w153) -> ("error out"=w156:errorcluster, "Profibus out"=w140:refnum<class "Profibus.lvclass">)  [unwired: 7 in]
                    }
                    frame Enabled {
                    }
                  }
                }
                frame "DeviceNET" {
                  n55 = disable-structure shown="Disabled" {
                    disable-tunnel: w167 -> [w181 _]
                    disable-tunnel: [w180 _] -> w166
                    disable-tunnel: [w179 _] -> w165
                    disable-tunnel: w164 -> [w173 _]
                    disable-tunnel: w163 -> [w169 _]
                    disable-tunnel: w162 -> [w168 _]
                    frame Disabled {
                      n56 = To More Specific Class(target class=refnum<class "DeviceNET.lvclass"> refnum ("DeviceNET.lvclass"), reference=w181) -> (specific class reference=w170:refnum<class "DeviceNET.lvclass">)  [unwired: 1 in, 1 out]
                      n57 = call-dynamic "Write DeviceNet Parameters.vi"("error in (no error)"=w173, "DeviceNet Interface Configuration"="DeviceNet Interface Configuration", "DeviceNET in"=w170) -> ("error out"=w172:errorcluster, "DeviceNET out"=w177:refnum<class "DeviceNET.lvclass">)  [unwired: 7 in]
                      n58 = call-dynamic "Write Interface Name.vi"("error in (no error)"=w172, "Interface Name"="Interface Name", "DeviceNET in"=w177) -> ("error out"=w171:errorcluster, "DeviceNET out"=w176:refnum<class "DeviceNET.lvclass">)  [unwired: 7 in]
                      n59 = call-dynamic "Setup.vi"("protocol selection ref"=w168, "error in (no error)"=w171, "Comm master cluster in"=w169, "DeviceNET in"=w176) -> ("error out"=w179:errorcluster, "DeviceNET out"=w180:refnum<class "DeviceNET.lvclass">)  [unwired: 6 in]
                    }
                    frame Enabled {
                    }
                  }
                }
              }
            }
            n60 = Bundle By Name(cluster=w70, "Read Complete?"=FALSE, "ProtocolRef"=w62, "ProtocolArray"=w68) -> (w69:T15)
          }
          frame "Read-Protocol" {
            # "Next state"
            # "Read-Protocol state - Reads selection"
            n61 = Unbundle By Name(w189) -> ("ProtocolArray"=w188:refnum<class "Protocol.lvclass">[], "ProtocolRef"=w187:refnum<vi>)
            n62 = Get Date/Time In Seconds() -> (seconds since 1Jan1904=w185:timestamp)
            n63 = Index Array(array="Protocol selection\n(appended)") -> (element=w192:T4)  [unwired: 1 in]
            n64 = Unbundle By Name(w192) -> ("Mode"=w191:T5)
            n65 = Format Date/Time String(time format string (%c)="%H:%M:%S %m.%d.%y", seconds (now)=w185) -> (date/time string=→"Test date and time":string)  [unwired: 1 in]
            n66 = call "convert_mode_index_to_enum.vi"("index"=w191, "CtlRef"=w187) -> ("Protocol enum"=w190:T20)  [unwired: 6 in, 3 out]
            n67 = for {
              tunnel: w190 -> [w201]
              tunnel: w188 -> [w200] mode=indexing
              tunnel: [w198] -> w186
              stop <- w199 stop-if-true
              n68 = call-dynamic "Match_protocol.vi"("Protocol type"=w201, "Protocol in"=w200) -> ("Match"=w199:bool, "Protocol out"=w198:refnum<class "Protocol.lvclass">)  [unwired: 7 in, 1 out]
            }
            n69 = Enqueue Element(queue=w196, element=ctrlCollectInfoStates."Read-CommInfo" ("ctrlCollectInfoStates"), error in (no error)=w195) -> (error out=w194:errorcluster)  [unwired: 1 in, 2 out]
            n70 = Bundle By Name(cluster=w189, "Protocol"=w186) -> (w197:T15)
          }
          frame "Read-CommInfo" {
            # "Next state"
            # "Read-CommInfo state - Reads common variable definitions from comm_map.csv"
            n71 = call <vilib>:"Application Directory.vi"() -> ("Application Directory"=w214:path)
            n72 = Build Path(base path=w214, name or relative path="data") -> (appended path=w210:path)
            n73 = Build Path(base path=w210, name or relative path="comm_map.csv") -> (appended path=w212:path)
            n74 = call "read_comm_definition.vi"("file path (dialog if empty)"=w212) -> ("error out"=w209:errorcluster, "Comm variable definitions"=w206:T16[])  [unwired: 8 in, 1 out]
            n75 = case shown="Error" w209 {
              frame No Error {
              }
              frame Error {
                n76 = call "Display Message to User"() -> ()  [unwired: 10 in, 2 out]
              }
            }
            n77 = Enqueue Element(queue=w205, element=ctrlCollectInfoStates."Read-ByteOrder" ("ctrlCollectInfoStates"), error in (no error)=w204) -> (error out=w203:errorcluster)  [unwired: 1 in, 2 out]
            n78 = Bundle By Name(cluster=w208, "Comm variable definitions"=w206) -> (w207:T15)
          }
          frame "Read-ByteOrder" {
            # "First read the byte order."
            # "Next state"
            # "Read-ByteOrder state - Reads Byte order"
            n79 = Unbundle By Name(w218) -> ("Comm variable definitions"=w219:T16[], "Protocol"=w220:refnum<class "Protocol.lvclass">)
            n80 = call "Search_comm_map_and_interrogate.vi"("array of registers"=w219, "Register name"="Byte order", "Protocol in"=w220) -> ("output cluster"=w222:T22)  [unwired: 6 in, 2 out]
            n81 = Unbundle By Name(w222) -> ("U16"=w221:u16)
            n82 = Type Cast(type=T2."2-3-0-1" ("Byte order"), x=w221) -> (*(type *) &x=w216:T2)
            "Byte order" <- w216
            n83 = Enqueue Element(queue=w227, element=ctrlCollectInfoStates."Read-FlowTubeMaterial" ("ctrlCollectInfoStates"), error in (no error)=w226) -> (error out=w225:errorcluster)  [unwired: 1 in, 2 out]
            n84 = Bundle By Name(cluster=w218, "Byte order"=w216) -> (w217:T15)
          }
          frame "Read-FlowTubeMaterial" {
            # "Next state"
            # "Read-FlowTubeMaterial state - Reads Flow Tube Material"
            n85 = Unbundle By Name(w235) -> ("Comm variable definitions"=w229:T16[], "Protocol"=w231:refnum<class "Protocol.lvclass">)
            n86 = call "Search_comm_map_and_interrogate.vi"("array of registers"=w229, "Register name"="Flow tube material", "Protocol in"=w231) -> ("output cluster"=w232:T22)  [unwired: 6 in, 2 out]
            n87 = Unbundle By Name(w232) -> ("U16"=w234:u16)
            "Flow Tube Material" <- w234
            n88 = flat-sequence {
              tunnel: [w240] -> w230
              tunnel: w234 -> [_]
              frame #0 {
                n89 = property on="Flow Tube Material" class="Ring (strict)"() -> ("RingText.Text"=w240:string)  [unwired: 2 in, 2 out]
              }
            }
            n90 = Enqueue Element(queue=w238, element=ctrlCollectInfoStates."Read-FlowCalibFactor" ("ctrlCollectInfoStates"), error in (no error)=w237) -> (error out=w236:errorcluster)  [unwired: 1 in, 2 out]
            n91 = Bundle By Name(cluster=w235, "Information.Material,9"=w230) -> (w239:T15)
          }
          frame "Read-FlowCalibFactor" {
            # "Next state"
            # "Read-FlowCalibFactor state - Reads Flow Calibration Factor"
            n92 = Unbundle By Name(w248) -> ("Comm variable definitions"=w243:T16[], "Protocol"=w242:refnum<class "Protocol.lvclass">)
            n93 = call "Search_comm_map_and_interrogate.vi"("array of registers"=w243, "Register name"="Flow Calibration Factor", "Protocol in"=w242) -> ("output cluster"=w246:T22)  [unwired: 6 in, 2 out]
            n94 = Unbundle By Name(w246) -> ("float"=w245:sgl)
            n95 = Number To Fractional String(number=w245) -> (F-format string=w244:string)  [unwired: 3 in]
            "FCF" <- w244
            n96 = Enqueue Element(queue=w251, element=ctrlCollectInfoStates."Read-D1" ("ctrlCollectInfoStates"), error in (no error)=w250) -> (error out=w249:errorcluster)  [unwired: 1 in, 2 out]
            n97 = Bundle By Name(cluster=w248, "Information.FCF, 14"=w244) -> (w252:T15)
          }
          frame "Read-D1" {
            # "Next state"
            # "Read-D1 state - Reads D1"
            n98 = Unbundle By Name(w260) -> ("Comm variable definitions"=w256:T16[], "Protocol"=w255:refnum<class "Protocol.lvclass">)
            n99 = call "Search_comm_map_and_interrogate.vi"("array of registers"=w256, "Register name"="D1", "Protocol in"=w255) -> ("output cluster"=w257:T22)  [unwired: 6 in, 2 out]
            n100 = Unbundle By Name(w257) -> ("float"=w258:sgl)
            n101 = Number To Fractional String(number=w258) -> (F-format string=w254:string)  [unwired: 3 in]
            "D1" <- w254
            n102 = Enqueue Element(queue=w263, element=ctrlCollectInfoStates."Read-D2" ("ctrlCollectInfoStates"), error in (no error)=w262) -> (error out=w261:errorcluster)  [unwired: 1 in, 2 out]
            n103 = Bundle By Name(cluster=w260, "Information.D1, 15"=w254) -> (w264:T15)
          }
          frame "Read-D2" {
            # "Next state"
            # "Read-D2 state - Reads D2"
            n104 = Unbundle By Name(w272) -> ("Comm variable definitions"=w268:T16[], "Protocol"=w267:refnum<class "Protocol.lvclass">)
            n105 = call "Search_comm_map_and_interrogate.vi"("array of registers"=w268, "Register name"="D2", "Protocol in"=w267) -> ("output cluster"=w269:T22)  [unwired: 6 in, 2 out]
            n106 = Unbundle By Name(w269) -> ("float"=w270:sgl)
            n107 = Number To Fractional String(number=w270) -> (F-format string=w266:string)  [unwired: 3 in]
            "D2" <- w266
            n108 = Enqueue Element(queue=w275, element=ctrlCollectInfoStates."Read-K1" ("ctrlCollectInfoStates"), error in (no error)=w274) -> (error out=w273:errorcluster)  [unwired: 1 in, 2 out]
            n109 = Bundle By Name(cluster=w272, "Information.D2, 16"=w266) -> (w276:T15)
          }
          frame "Read-K1" {
            # "Next state"
            # "Read-K1 state - Reads K1"
            n110 = Unbundle By Name(w284) -> ("Comm variable definitions"=w280:T16[], "Protocol"=w279:refnum<class "Protocol.lvclass">)
            n111 = call "Search_comm_map_and_interrogate.vi"("array of registers"=w280, "Register name"="K1", "Protocol in"=w279) -> ("output cluster"=w282:T22)  [unwired: 6 in, 2 out]
            n112 = Unbundle By Name(w282) -> ("float"=w283:sgl)
            n113 = Number To Fractional String(number=w283) -> (F-format string=w278:string)  [unwired: 3 in]
            "K1" <- w278
            n114 = Enqueue Element(queue=w287, element=ctrlCollectInfoStates."Read-K2" ("ctrlCollectInfoStates"), error in (no error)=w286) -> (error out=w285:errorcluster)  [unwired: 1 in, 2 out]
            n115 = Bundle By Name(cluster=w284, "Information.K1, 17"=w278) -> (w288:T15)
          }
          frame "Read-K2" {
            # "Next state"
            # "Read-K2 state - Reads K2"
            n116 = Unbundle By Name(w296) -> ("Comm variable definitions"=w291:T16[], "Protocol"=w290:refnum<class "Protocol.lvclass">)
            n117 = call "Search_comm_map_and_interrogate.vi"("array of registers"=w291, "Register name"="K2", "Protocol in"=w290) -> ("output cluster"=w293:T22)  [unwired: 6 in, 2 out]
            n118 = Unbundle By Name(w293) -> ("float"=w294:sgl)
            n119 = Number To Fractional String(number=w294) -> (F-format string=w292:string)  [unwired: 3 in]
            "K2" <- w292
            n120 = Enqueue Element(queue=w299, element=ctrlCollectInfoStates."Read-FD" ("ctrlCollectInfoStates"), error in (no error)=w298) -> (error out=w297:errorcluster)  [unwired: 1 in, 2 out]
            n121 = Bundle By Name(cluster=w296, "Information.K2, 18"=w292) -> (w300:T15)
          }
          frame "Read-FD" {
            # "Next state"
            # "Read-FD state - Reads FD"
            n122 = Unbundle By Name(w308) -> ("Comm variable definitions"=w304:T16[], "Protocol"=w303:refnum<class "Protocol.lvclass">)
            n123 = call "Search_comm_map_and_interrogate.vi"("array of registers"=w304, "Register name"="FD", "Protocol in"=w303) -> ("output cluster"=w307:T22)  [unwired: 6 in, 2 out]
            n124 = Unbundle By Name(w307) -> ("float"=w305:sgl)
            n125 = Number To Fractional String(number=w305) -> (F-format string=w302:string)  [unwired: 3 in]
            "FD" <- w302
            n126 = Enqueue Element(queue=w311, element=ctrlCollectInfoStates."Read-DenTempCoeff" ("ctrlCollectInfoStates"), error in (no error)=w310) -> (error out=w309:errorcluster)  [unwired: 1 in, 2 out]
            n127 = Bundle By Name(cluster=w308, "Information.FD, 19"=w302) -> (w312:T15)
          }
          frame "Read-DenTempCoeff" {
            # "Next state"
            # "Read-DenTempCoeff state - Reads Density Temperature Coefficient"
            n128 = Unbundle By Name(w320) -> ("Comm variable definitions"=w315:T16[], "Protocol"=w314:refnum<class "Protocol.lvclass">)
            n129 = call "Search_comm_map_and_interrogate.vi"("array of registers"=w315, "Register name"="Density Temperature Coefficient", "Protocol in"=w314) -> ("output cluster"=w317:T22)  [unwired: 6 in, 2 out]
            n130 = Unbundle By Name(w317) -> ("float"=w318:sgl)
            n131 = Number To Fractional String(number=w318) -> (F-format string=w316:string)  [unwired: 3 in]
            "Density Temp Coeff" <- w316
            n132 = Bundle By Name(cluster=w320, "Information.Density Temp Coeff, 20"=w316) -> (w324:T15)
            n133 = Enqueue Element(queue=w323, element=ctrlCollectInfoStates."Read-Srno" ("ctrlCollectInfoStates"), error in (no error)=w322) -> (error out=w321:errorcluster)  [unwired: 1 in, 2 out]
          }
          frame "Read-Srno" {
            # "Next state"
            # "Read-Srno state -  Reads Serial Number"
            n134 = Unbundle By Name(w332) -> ("Comm variable definitions"=w327:T16[], "Protocol"=w326:refnum<class "Protocol.lvclass">)
            n135 = call "Search_comm_map_and_interrogate.vi"("array of registers"=w327, "Register name"="Serial Number", "Protocol in"=w326) -> ("output cluster"=w330:T22)  [unwired: 6 in, 2 out]
            n136 = Unbundle By Name(w330) -> ("U32"=w329:u32)
            n137 = Number To Decimal String(number=w329) -> (decimal integer string=w328:string)  [unwired: 1 in]
            "Sensor Serial Number" <- w328
            n138 = Bundle By Name(cluster=w332, "Information.Transmitter Serial Number,23"=w328) -> (w336:T15)
            n139 = Enqueue Element(queue=w335, element=ctrlCollectInfoStates."Read-MassFlowUnits" ("ctrlCollectInfoStates"), error in (no error)=w334) -> (error out=w333:errorcluster)  [unwired: 1 in, 2 out]
          }
          frame "Read-MassFlowUnits" {
            # "Next state"
            # "Read-MassFlowUnits state - Reads Mass flow units"
            n140 = Unbundle By Name(w344) -> ("Comm variable definitions"=w340:T16[], "Protocol"=w339:refnum<class "Protocol.lvclass">)
            n141 = call "Search_comm_map_and_interrogate.vi"("array of registers"=w340, "Register name"="Mass flow units", "Protocol in"=w339) -> ("output cluster"=w342:T22)  [unwired: 6 in, 2 out]
            n142 = Unbundle By Name(w342) -> ("U16"=w341:u16)
            "Mass flow units" <- w341
            n143 = flat-sequence {
              tunnel: [w349] -> w338
              tunnel: w341 -> [_]
              frame #0 {
                n144 = property on="Mass flow units" class="Ring (strict)"() -> ("RingText.Text"=w349:string)  [unwired: 2 in, 2 out]
              }
            }
            n145 = Enqueue Element(queue=w347, element=ctrlCollectInfoStates."Read-DensityUnits" ("ctrlCollectInfoStates"), error in (no error)=w346) -> (error out=w345:errorcluster)  [unwired: 1 in, 2 out]
            n146 = Bundle By Name(cluster=w344, "Information.Mass Flow Units, 25"=w338) -> (w348:T15)
          }
          frame "Read-DensityUnits" {
            # "Next state"
            # "Read-DensityUnits state - Reads Density units"
            n147 = Unbundle By Name(w357) -> ("Comm variable definitions"=w353:T16[], "Protocol"=w352:refnum<class "Protocol.lvclass">)
            n148 = call "Search_comm_map_and_interrogate.vi"("array of registers"=w353, "Register name"="Density units", "Protocol in"=w352) -> ("output cluster"=w355:T22)  [unwired: 6 in, 2 out]
            n149 = Unbundle By Name(w355) -> ("U16"=w354:u16)
            "Density units" <- w354
            n150 = flat-sequence {
              tunnel: [w362] -> w351
              tunnel: w354 -> [_]
              frame #0 {
                n151 = property on="Density units" class="Ring (strict)"() -> ("RingText.Text"=w362:string)  [unwired: 2 in, 2 out]
              }
            }
            n152 = Enqueue Element(queue=w360, element=ctrlCollectInfoStates."Read-TempUnits" ("ctrlCollectInfoStates"), error in (no error)=w359) -> (error out=w358:errorcluster)  [unwired: 1 in, 2 out]
            n153 = Bundle By Name(cluster=w357, "Information.Density Units, 26"=w351) -> (w361:T15)
          }
          frame "Read-TempUnits" {
            # "Next state"
            # "Read-TempUnits state - Reads Temperature units"
            n154 = Unbundle By Name(w370) -> ("Comm variable definitions"=w366:T16[], "Protocol"=w365:refnum<class "Protocol.lvclass">)
            n155 = call "Search_comm_map_and_interrogate.vi"("array of registers"=w366, "Register name"="Temperature units", "Protocol in"=w365) -> ("output cluster"=w368:T22)  [unwired: 6 in, 2 out]
            n156 = Unbundle By Name(w368) -> ("U16"=w367:u16)
            "Temperature Units" <- w367
            n157 = flat-sequence {
              tunnel: [w375] -> w364
              tunnel: w367 -> [_]
              frame #0 {
                n158 = property on="Temperature Units" class="Ring (strict)"() -> ("RingText.Text"=w375:string)  [unwired: 2 in, 2 out]
              }
            }
            n159 = Enqueue Element(queue=w373, element=ctrlCollectInfoStates."Read-FlowCutoff" ("ctrlCollectInfoStates"), error in (no error)=w372) -> (error out=w371:errorcluster)  [unwired: 1 in, 2 out]
            n160 = Bundle By Name(cluster=w370, "Information.Temperature Units, 27"=w364) -> (w374:T15)
          }
          frame "Read-FlowCutoff" {
            # "Next state"
            # "Read-FlowCutoff state - Reads Mass flow cutoff"
            n161 = Unbundle By Name(w383) -> ("Comm variable definitions"=w379:T16[], "Protocol"=w378:refnum<class "Protocol.lvclass">)
            n162 = call "Search_comm_map_and_interrogate.vi"("array of registers"=w379, "Register name"="Mass flow cutoff", "Protocol in"=w378) -> ("output cluster"=w381:T22)  [unwired: 6 in, 2 out]
            n163 = Unbundle By Name(w381) -> ("float"=w380:sgl)
            n164 = Number To Fractional String(number=w380) -> (F-format string=w377:string)  [unwired: 3 in]
            "Mass flow cutoff" <- w377
            n165 = Enqueue Element(queue=w386, element=ctrlCollectInfoStates."Read-MassFlowDamping" ("ctrlCollectInfoStates"), error in (no error)=w385) -> (error out=w384:errorcluster)  [unwired: 1 in, 2 out]
            n166 = Bundle By Name(cluster=w383, "Information.Mass Flow Cutoff, 28"=w377) -> (w387:T15)
          }
          frame "Read-MassFlowDamping" {
            # "Next state"
            # "Read-MassFlowDamping state - Reads Flow rate internal damping"
            n167 = Unbundle By Name(w395) -> ("Comm variable definitions"=w390:T16[], "Protocol"=w389:refnum<class "Protocol.lvclass">)
            n168 = call "Search_comm_map_and_interrogate.vi"("array of registers"=w390, "Register name"="Flow rate internal damping", "Protocol in"=w389) -> ("output cluster"=w393:T22)  [unwired: 6 in, 2 out]
            n169 = Unbundle By Name(w393) -> ("float"=w392:sgl)
            n170 = Number To Fractional String(number=w392) -> (F-format string=w391:string)  [unwired: 3 in]
            "Mass flow damping" <- w391
            n171 = Bundle By Name(cluster=w395, "Information.Mass Flow Damping, 29"=w391) -> (w399:T15)
            n172 = Enqueue Element(queue=w398, element=ctrlCollectInfoStates."Read-FlowDirection" ("ctrlCollectInfoStates"), error in (no error)=w397) -> (error out=w396:errorcluster)  [unwired: 1 in, 2 out]
          }
          frame "Read-FlowDirection" {
            # "Next state"
            # "Read-FlowDirection state - Reads Flow direction"
            n173 = Unbundle By Name(w407) -> ("Comm variable definitions"=w403:T16[], "Protocol"=w402:refnum<class "Protocol.lvclass">)
            n174 = call "Search_comm_map_and_interrogate.vi"("array of registers"=w403, "Register name"="Flow direction", "Protocol in"=w402) -> ("output cluster"=w405:T22)  [unwired: 6 in, 2 out]
            n175 = Unbundle By Name(w405) -> ("U16"=w404:u16)
            "Flow direction" <- w404
            n176 = flat-sequence {
              tunnel: w404 -> [_]
              tunnel: [w412] -> w401
              frame #0 {
                n177 = property on="Flow direction" class="Ring (strict)"() -> ("RingText.Text"=w412:string)  [unwired: 2 in, 2 out]
              }
            }
            n178 = Enqueue Element(queue=w410, element=ctrlCollectInfoStates."Read-FreqFlowRate" ("ctrlCollectInfoStates"), error in (no error)=w409) -> (error out=w408:errorcluster)  [unwired: 1 in, 2 out]
            n179 = Bundle By Name(cluster=w407, "Information.Flow Direction, 30"=w401) -> (w411:T15)
          }
          frame "Read-FreqFlowRate" {
            # "Next state"
            # "Read-FreqFlowRate state - Reads Frequency/pulse output present frequency"
            n180 = Unbundle By Name(w420) -> ("Comm variable definitions"=w416:T16[], "Protocol"=w415:refnum<class "Protocol.lvclass">)
            n181 = call "Search_comm_map_and_interrogate.vi"("array of registers"=w416, "Register name"="Frequency/pulse output present frequency", "Protocol in"=w415) -> ("output cluster"=w418:T22)  [unwired: 6 in, 2 out]
            n182 = Unbundle By Name(w418) -> ("float"=w417:sgl)
            n183 = Number To Fractional String(number=w417) -> (F-format string=w414:string)  [unwired: 3 in]
            "Frequency flow rate" <- w414
            n184 = Bundle By Name(cluster=w420, "Information.Frequency Flow Rate, 31"=w414) -> (w424:T15)
            n185 = Enqueue Element(queue=w423, element=ctrlCollectInfoStates."Read-FreqSpan" ("ctrlCollectInfoStates"), error in (no error)=w422) -> (error out=w421:errorcluster)  [unwired: 1 in, 2 out]
          }
          frame "Read-FreqSpan" {
            # "Next state"
            # "Read-FreqSpan state - Reads Frequency maximum pulse width"
            n186 = Unbundle By Name(w432) -> ("Comm variable definitions"=w427:T16[], "Protocol"=w426:refnum<class "Protocol.lvclass">)
            n187 = call "Search_comm_map_and_interrogate.vi"("array of registers"=w427, "Register name"="Frequency maximum pulse width ", "Protocol in"=w426) -> ("output cluster"=w430:T22)  [unwired: 6 in, 2 out]
            n188 = Unbundle By Name(w430) -> ("float"=w429:sgl)
            n189 = Number To Fractional String(number=w429) -> (F-format string=w428:string)  [unwired: 3 in]
            "Frequency span" <- w428
            n190 = Enqueue Element(queue=w435, element=ctrlCollectInfoStates."Read-TransmitterModel" ("ctrlCollectInfoStates"), error in (no error)=w434) -> (error out=w433:errorcluster)  [unwired: 1 in, 2 out]
            n191 = Bundle By Name(cluster=w432, "Information.Frequency Span, 32"=w428) -> (w436:T15)
          }
          frame "Read-TransmitterModel" {
            # "Next state"
            # "Read-TransmitterModel state - Reads Transmitter model"
            n192 = Unbundle By Name(w444) -> ("Comm variable definitions"=w439:T16[], "Protocol"=w438:refnum<class "Protocol.lvclass">)
            n193 = call "Search_comm_map_and_interrogate.vi"("array of registers"=w439, "Register name"="Transmitter model", "Protocol in"=w438) -> ("output cluster"=w442:T22)  [unwired: 6 in, 2 out]
            n194 = Unbundle By Name(w442) -> ("U16"=w441:u16)
            n195 = Number To Decimal String(number=w441) -> (decimal integer string=w440:string)  [unwired: 1 in]
            "Transmitter Model" <- w440
            n196 = Bundle By Name(cluster=w444, "Information.Transmitter Model Number,24"=w440) -> (w448:T15)
            n197 = Enqueue Element(queue=w447, element=ctrlCollectInfoStates."Read-MeterZero" ("ctrlCollectInfoStates"), error in (no error)=w446) -> (error out=w445:errorcluster)  [unwired: 1 in, 2 out]
          }
          frame "Read-MeterZero" {
            # "Next state"
            # "Read-MeterZero state - Reads MeterZero"
            n198 = Unbundle By Name(w457) -> ("Comm variable definitions"=w451:T16[], "Protocol"=w450:refnum<class "Protocol.lvclass">)
            n199 = call "Search_comm_map_and_interrogate.vi"("array of registers"=w451, "Register name"="Meter Zero", "Protocol in"=w450) -> ("error out"=w456:errorcluster, "output cluster"=w453:T22)  [unwired: 6 in, 1 out]
            n200 = Unbundle By Name(w456) -> ("status"=→"status":bool)
            n201 = Unbundle By Name(w453) -> ("float"=w452:sgl)
            n202 = Number To Fractional String(number=w452) -> (F-format string=w449:string)  [unwired: 3 in]
            "Meter Zero" <- w449
            n203 = Enqueue Element(queue=w461, element=ctrlCollectInfoStates."ReadComplete" ("ctrlCollectInfoStates"), error in (no error)=w460) -> (error out=w459:errorcluster)  [unwired: 1 in, 2 out]
            n204 = Bundle By Name(cluster=w457, "Information.Meter Zero, 43"=w449) -> (w462:T15)
          }
          frame "ReadComplete" {
            # "Next state"
            # "ReadComplete state - Update Read Complete? status"
            n205 = Enqueue Element(queue=w468, element=ctrlCollectInfoStates."WaitforEvents" ("ctrlCollectInfoStates"), error in (no error)=w467) -> (error out=w466:errorcluster)  [unwired: 1 in, 2 out]
            n206 = Bundle By Name(cluster=w464, "Read Complete?"=TRUE) -> (w469:T15)
          }
          frame "Done&Close" {
            # "Done&Close state - Updates output"
            n207 = Unbundle By Name(w474) -> ("Read Complete?"=→"Read Completed":bool, "Information"=w475:T9)
            n208 = Equal?(x="Status *", y=enum32{"As found", "As left"}."As found") -> (x = y?=w488:bool)
            n209 = Select(t="As found" ("Technician Name*"), s=w488, f="As left") -> (s? t:f=w479:string)
            n210 = Bundle By Name(cluster=w475, "Test Comments,3"="Test Comments", "Transmitter Serial Number,23"="Transmitter Serial Number", "Sensor Model,7"="Sensor Model #", "Size,8"="Size", "Press rating, 10"="Pressure Rating", "Temp rating, 11"="Temp Rating", "Flow Accuracy, 35"="Meter flow accuracy (%) *", "Flow Repeatability, 36"="Meter flow repeatability", "Zero Stability, 37"="Meter Zero Stability (kg/min) *", "Density Accuracy, 38"="Meter Density Accuracy", "Density Repeatability, 39"="Meter Density Repeatability", "Nomincal Flow Rate, 41"="Meter Nominal Flow Rate (kg/min)*", "Customer name, 46"="Customer Name", "Customer address, 47"="Customer Address", "Sales order number, 48"="Order number", "Technician Name, 49"="Technician Name*", "ref meter, 50"="Ref meter serial number*", "Status, 45"=w479, "product code,51"="Product code*", "fluid,52"="Fluid") -> (w472:T9)
            "Information" <- w472
            n211 = Bundle By Name(cluster=w474, "Information"=w472) -> (w473:T15)
          }
        }
      }
      frame Error {
        # "Clear errors..."
        # "Return true in any case that should stop the loop."
        n212 = call <vilib>:"Clear Errors.vi"("error in (no error)"=w503) -> ("error out"=w502:errorcluster)  [unwired: 5 in, 1 out]
      }
    }
  }
  n213 = Release Queue(queue=w4, error in (no error)=w5) -> (error out=w7:errorcluster)  [unwired: 1 in, 2 out]
  n214 = call <vilib>:"Clear Errors.vi"("error in (no error)"=w7) -> ()  [unwired: 5 in, 2 out]
